vi "Home Subvi.vi"(4 "error in (no error)":errorcluster, 6 "Only Z?":bool, 7 "controller in":refnum<k24>) -> (0 "error out":errorcluster, 3 "controller out":refnum<k24>)   [LabVIEW 2011]
uses:
  C:/Users/Admin/Desktop/Gantry Code Transfer/source/Code Transfer/Aerotech.A3200.dll
  Aerotech.A3200.dll
  WaitSingle.vi
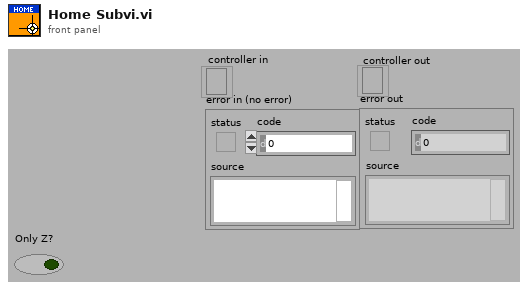
[diagram p1: front panel]
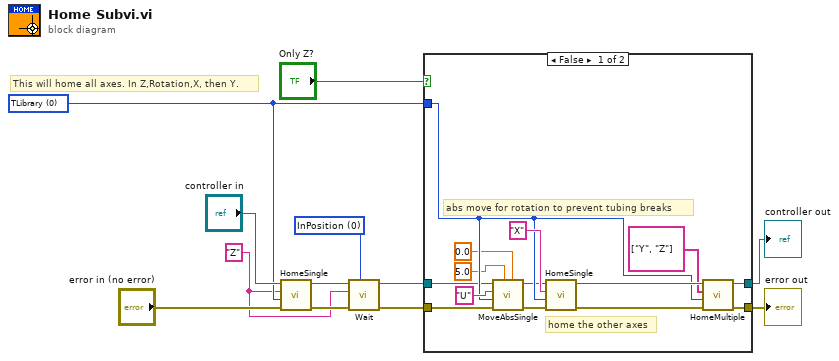
[diagram p0: block diagram]
diagram:
  w4 = 0 items=["InPosition", "MoveDone"] ("wait option?")
  w3 = "Z" ("axis name")
  w11 = 0 items=["TLibrary", "T01", "T02", "T03", "T04", "T05", "T06", "T07", "T08", "T09", "T10", "T11", "T12", "T13", "T14", "T15", "T16", "T17", "T18", "T19", "T20", "T21", "T22", "T23", "T24", "T25", "T26", "T27", "T28", "T29", "T30", "T31"] ("taskId")
  # "This will home all axes. In Z,Rotation,X, then Y."
  n1 = call "HomeSingle.vi"("error in (no error)"="error in (no error)", "taskId"=w11, "axis name"=w3, "controller in"="controller in") -> ("error out"=w5:errorcluster, "controller out"=w6:refnum<k24>)  [unwired: 6 in]
  n2 = call-poly "Wait.vi"("wait option?"=w4, "error in (no error)"=w5, "axis name"=w3, "controller in"=w6) -> ("error out"=w1:errorcluster, "controller out"=w2:refnum<k24>)  [unwired: 5 in, 1 out]
  n3 = case shown="False" "Only Z?" {
    tunnel: w11 -> [w22 _]
    tunnel: w2 -> [w21 w28]
    tunnel: w1 -> [w20 w27]
    tunnel: [w14 w27] -> w9
    tunnel: [w13 w28] -> w8
    frame False {
      # "abs move for rotation to prevent tubing breaks"
      # "home the other axes"
      n4 = call "MoveAbsSingle.vi"("position"=0.0, "speed"=5.0, "error in (no error)"=w20, "taskId"=w22, "axis name"="U", "controller in"=w21) -> ("error out"=w18:errorcluster, "controller out"=w19:refnum<k24>)  [unwired: 4 in]
      n5 = call "HomeSingle.vi"("error in (no error)"=w18, "taskId"=w22, "axis name"="X", "controller in"=w19) -> ("error out"=w24:errorcluster, "controller out"=w25:refnum<k24>)  [unwired: 6 in]
      n6 = call "HomeMultiple.vi"("error in (no error)"=w24, "taskId"=w22, "axis names"=string[] ["Y", "Z"], "controller in"=w25) -> ("error out"=w14:errorcluster, "controller out"=w13:refnum<k24>)  [unwired: 6 in]
    }
    frame True {
      # "do nothing else"
    }
  }
  "controller out" <- w8
  "error out" <- w9
